vi "AW_Calculate_Tester_Parameter.vi"(8 "Tester Parameter":dbl[](array[numeric]), 9 "DDM Parameter":dbl[](array[numeric]), 10 "AW_Box_Pressure/Stag Total-Static Pressure rise":dbl, 11 "Orifice_Plate_Diameter":dbl) -> (3 "Calculate Tester Parameter":dbl[](array[numeric]))   [LabVIEW 2017]
panel:
  out "Suction_Power_Rated_Power":dbl format="%#_6f"
  out "Volumetric_Flow_Rate_Rated_Power":dbl
  out "delta_v":dbl
  out "ddm_real_power":dbl
  out "DDM Pressure":dbl
  out "DDM Measured Power":dbl
  out "DDM Speed":dbl
  out "DDM Power":dbl
  out "DDM Current":dbl
  out "DDM Voltage":dbl
  out "Ambient humidity":dbl
  out "Ambient temperature":dbl
  out "Ambient pressure":dbl
  out "power":dbl
  out "current":dbl
  out "voltage":dbl
  out "DDM_Pressure_corrected":dbl
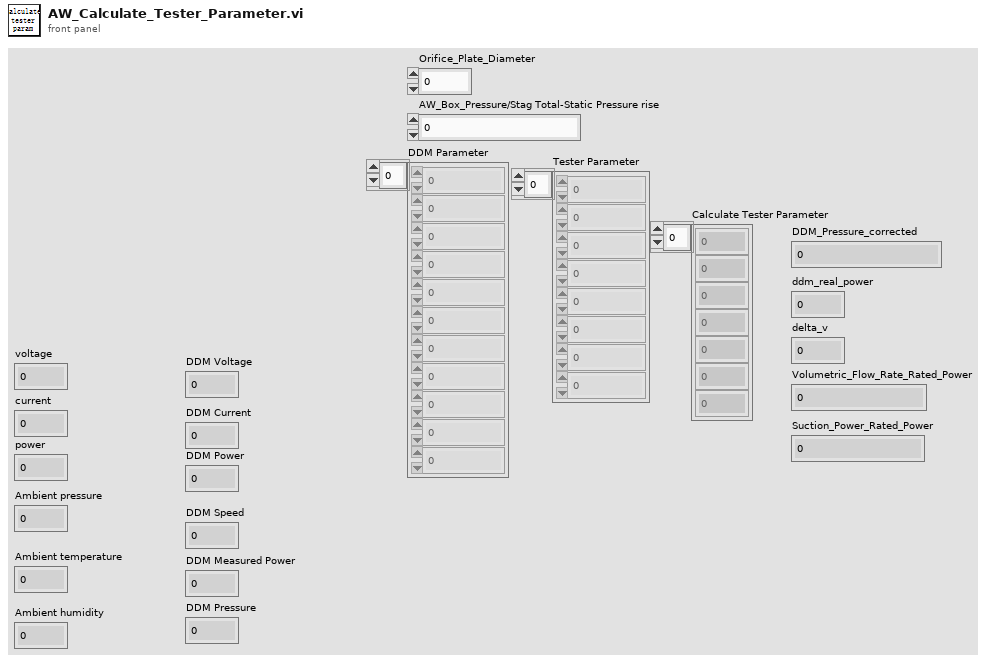
[diagram p1: front panel]
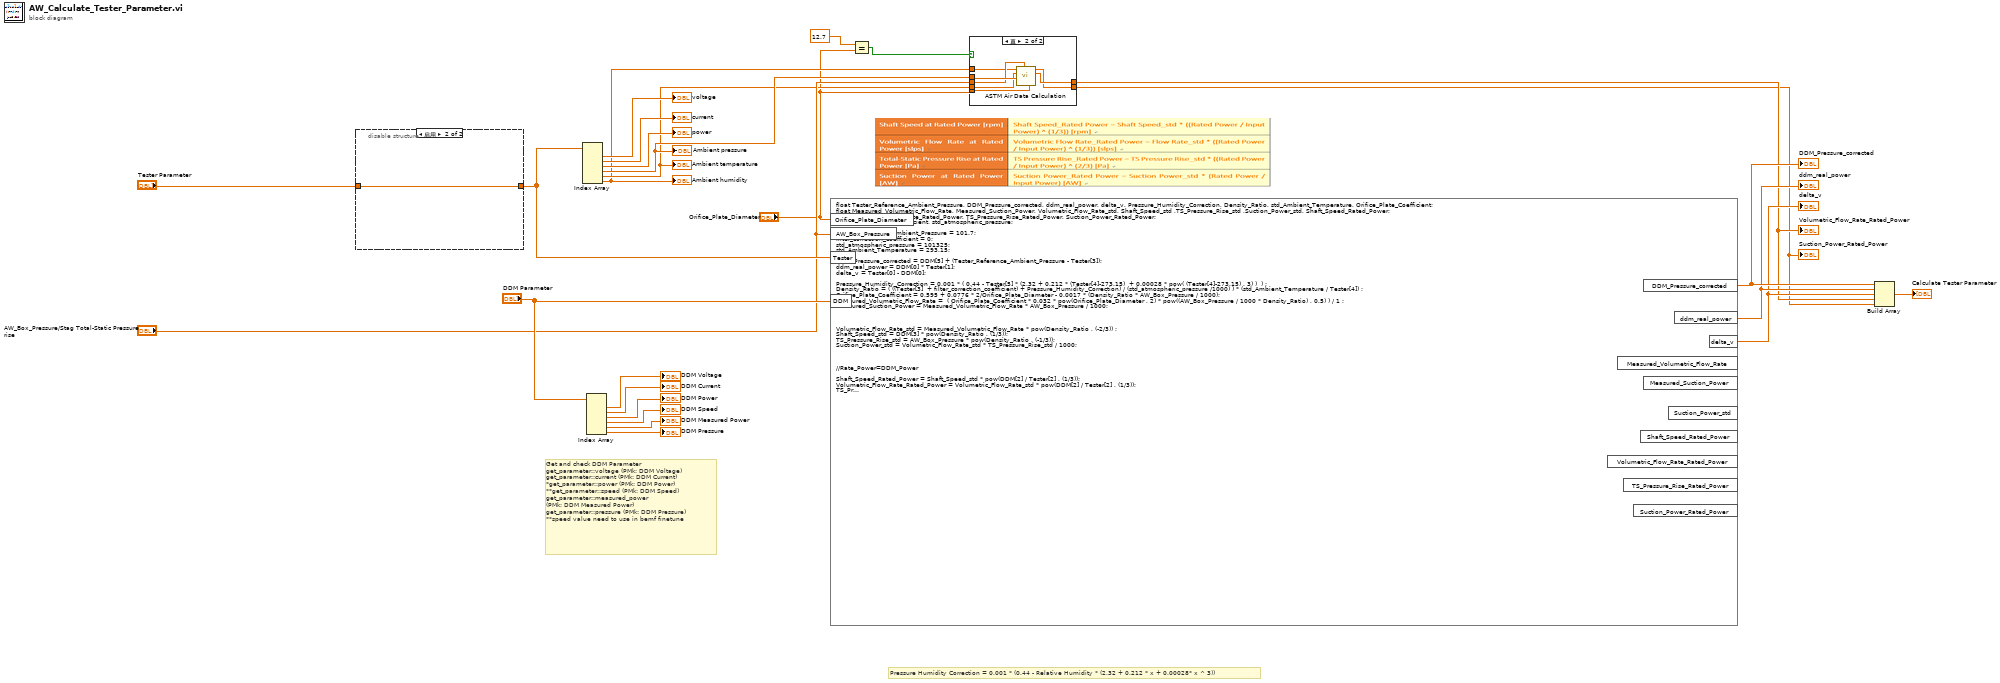
[diagram p0: block diagram]
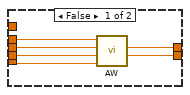
[diagram p2: hidden frame]
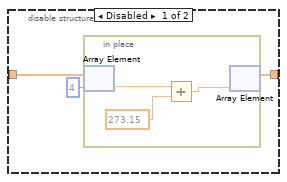
[diagram p3: hidden frame]
diagram:
  # "Pressure Humidity Correction = 0.001 * (0.44 - Relative Humidity * (2.32 + 0.212 * x + 0.00028* x ^ 3))"
  # "Get and check DDM Parameter\nget_parameter::voltage (PMk: DDM Voltage)\nget_parameter::current (PMk: DDM Current)\n*get_parameter::power (PMk: DDM Power)\n**get_parameter::speed (PMk: DDM Speed)\nget_parameter::measured_power\n(PMk: DDM Measured Power)\nget_parameter::pressure (PMk: DDM Pressure)\n**speed value need to use in bemf finetune"
  n1 = disable-structure shown="启用" {
    disable-tunnel: [w28 w32] -> w11
    disable-tunnel: "Tester Parameter" -> [w26 w32]
    frame Disabled {
      n2 = in-place {
        n3 = in-place-array #1(w26, 4) -> (w31:dbl)
        n4 = Add(x=w31, y=273.15) -> (x+y=w30:dbl)
        n5 = in-place-array #1(w30) -> (w28:dbl[])  [unwired: 1 out]
      }
    }
    frame Enabled {
    }
  }
  n6 = Index Array(array=w11) -> (element #1=→"voltage":dbl, element #2=→"current":dbl, element #3=→"power":dbl, element #4=w8:dbl, element #5=w7:dbl, element #6=w4:dbl)  [unwired: 6 in]
  "Ambient pressure" <- w8
  "Ambient temperature" <- w7
  "Ambient humidity" <- w4
  n7 = Index Array(array="DDM Parameter") -> (element #1=→"DDM Voltage":dbl, element #2=→"DDM Current":dbl, element #3=→"DDM Power":dbl, element #4=→"DDM Speed":dbl, element #5=→"DDM Measured Power":dbl, element #6=→"DDM Pressure":dbl)  [unwired: 6 in]
  n8 = formula code="float Tester_Reference_Ambient_Pressure, DDM_Pressure_corrected, ddm_real_power, delta_v, Pressure_Humidity_Correction, Density_Ratio, std_Ambient_Temperature, Orifice_Plate_Coefficient;\nfloat Measured_Volumetric_Flow_Rate, Measured_Suction_Power, Volumetric_Flow_Rate_std, Shaft_Speed_std ,TS_Pressure_Rise_std ,Suction_Power_std, Shaft_Speed_Rated_Power;\nfloat Volumetric_Flow_Rate_Rated_Power, TS_Pressure_Rise_Rated_Power, Suction_Power_Rated_Power;\nint filter_correction_coefficient, std_atmospheric_pressure;\n\nTester_Reference_Ambient_Pressure = 101.7;\nfilter_correction_coefficient = 0;\nstd_atmospheric_pressure = 101325;\nstd_Ambient_Temperature = 293.15;\n\nDDM_Pressure_corrected = DDM[5] + (Tester_Reference_Ambient_Pressure - Tester[3]);\nddm_real_power = DDM[0] * Tester[1];\ndelta_v = Tester[0] - DDM[0];\n\nPressure_Humidity_Correction = 0.001 * ( 0.44 - Tester[5] * (2.32 + 0.212 * (Tester[4]-273.15)  + 0.00028 * pow( (Tester[4]-273.15) , 3) )  ) ;\nDensity_Ratio = ( ((Tester[3]  + filter_correction_coefficient) + Pressure_Humidity_Correction) / (std_atmospheric_pressure /1000) ) * (std_Ambient_Temperature / Tester[4]) ;\nOrifice_Plate_Coefficient = 0.595 + 0.0776 * 2/Orifice_Plate_Diameter - 0.0017 * (Density_Ratio * AW_Box_Pressure / 1000);\nMeasured_Volumetric_Flow_Rate =  ( Orifice_Plate_Coefficient * 0.032 * pow(Orifice_Plate_Diameter , 2) * pow((AW_Box_Pressure / 1000 * Density_Ratio) , 0.5) ) / 1 ;\nMeasured_Suction_Power = Measured_Volumetric_Flow_Rate * AW_Box_Pressure / 1000;\n\n\n\nVolumetric_Flow_Rate_std = Measured_Volumetric_Flow_Rate * pow(Density_Ratio , (-2/3)) ;\nShaft_Speed_std = DDM[3] * pow(Density_Ratio , (1/3));\nTS_Pressure_Rise_std = AW_Box_Pressure * pow(Density_Ratio , (-1/3));\nSuction_Power_std = Volumetric_Flow_Rate_std * TS_Pressure_Rise_std / 1000;\n\n\n\n//Rate_Power=DDM_Power\n\nShaft_Speed_Rated_Power = Shaft_Speed_std * pow(DDM[2] / Tester[2] , (1/3));\nVolumetric_Flow_Rate_Rated_Power = Volumetric_Flow_Rate_std * pow(DDM[2] / Tester[2] , (1/3));\nTS_Pressure_Rise_Rated_Power = TS_Pressure_Rise_std * pow(DDM[2] / Tester[2] , (2/3));\nSuction_Power_Rated_Power = Suction_Power_std * (DDM[2] / Tester[2]);"("Tester"=w11, "DDM"="DDM Parameter", "Orifice_Plate_Diameter"="Orifice_Plate_Diameter", "AW_Box_Pressure"="AW_Box_Pressure/Stag Total-Static Pressure rise") -> ("DDM_Pressure_corrected"=w15:dbl, "ddm_real_power"=w14:dbl, "delta_v"=w13:dbl)  [unwired: 7 out]
  "DDM_Pressure_corrected" <- w15
  "ddm_real_power" <- w14
  "delta_v" <- w13
  n9 = Equal?(x=12.7, y="Orifice_Plate_Diameter") -> (x = y?=w1:bool)
  n10 = case shown="真" w1 {
    tunnel: "Orifice_Plate_Diameter" -> [w38 w43]
    tunnel: "AW_Box_Pressure/Stag Total-Static Pressure rise" -> [w37 w40]
    tunnel: w8 -> [w36 w42]
    tunnel: w7 -> [w35 w41]
    tunnel: [w34 w45] -> w6
    tunnel: [w33 w44] -> w5
    tunnel: w4 -> [_ w39]
    frame False {
      n11 = call "AW.vi"("Orifice_Plate_Diameter"=w38, "Ambient_temperature"=w35, "Box_Pressure"=w37, "Ambient_Pressure"=w36) -> ("AP"=w33:dbl, "Q"=w34:dbl)  [unwired: 6 in]
    }
    frame True {
      n12 = call "ASTM Air Data Calculation.vi"("Orifice (mm)"=w43, "Suction Pressure (kPa)"=w40, "Ambient Pressure (kPa) Bt"=w42, "Ambient Temperature (C)"=w41, "Ambient Humudity (%)"=w39) -> ("Flow-Rate (l/s), Q"=w45:dbl, "Suction Power in Air Watt"=w44:dbl)  [unwired: 4 in, 1 out]
    }
  }
  "Volumetric_Flow_Rate_Rated_Power" <- w6
  "Suction_Power_Rated_Power" <- w5
  n13 = Build Array(w15, w14, w13, w6, w5) -> (→"Calculate Tester Parameter":dbl[])
